vi "Periodic Tasks.vi"(8 "error in":errorcluster) -> ()   [LabVIEW 2017]
doc: "This VI runs in parallel to other tasks. It can contain as many user-defined periodic loops as you need. These can carry out PID or other sorts of timed response."
uses:
  Team-code/IntakeSubsystem.vi
  Team-code/CubeLiftSubsystem.vi
  Team-code/RobotLiftSubsystem.vi
  Team-code/DriveSubsystem.vi
  labview-standard-library/data-logging.lvlib
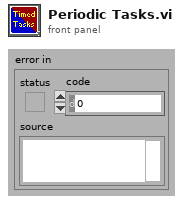
[diagram p1: front panel]
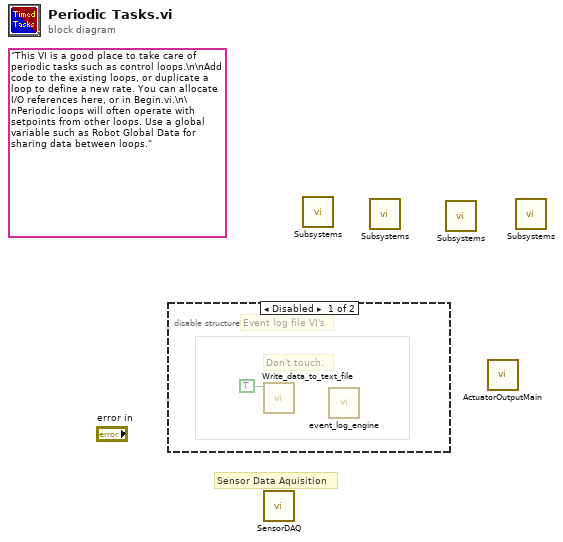
[diagram p0: block diagram]
diagram:
  (unwired) "This VI is a good place to take care of periodic tasks such as control loops.\n\nAdd code to the existing loops, or duplicate a loop to define a new rate. You can allocate I/O references here, or in Begin.vi.\n\nPeriodic loops will often operate with setpoints from other loops. Use a global variable such as Robot Global Data for sharing data between loops."
  # "Sensor Data Aquisition"
  n1 = disable-structure shown="Disabled" {
    frame Disabled {
      # "Don't touch."
      # "Event log file VI's"
      n2 = call "Write_data_to_text_file.vi"(".CSV? (F=.txt)"=TRUE) -> ()  [unwired: 11 in]
      n3 = call "event_log_engine.vi"() -> ()  [unwired: 10 in, 2 out]
    }
    frame Enabled {
    }
  }
  n4 = call "SensorDAQ.vi"() -> ()  [unwired: 12 in]
  n5 = call-poly "Subsystems.vi"() -> ()  [unwired: 12 in]
  n6 = call-poly "Subsystems.vi"() -> ()  [unwired: 12 in]
  n7 = call-poly "Subsystems.vi"() -> ()  [unwired: 12 in]
  n8 = call "ActuatorOutputMain.vi"() -> ()  [unwired: 12 in]
  n9 = call-poly "Subsystems.vi"() -> ()  [unwired: 12 in]
